vi "click_sp_coord.vi"(8 "error in (no error)":errorcluster, 10 "Panel":refnum<vi>, 11 "SubPanel in":refnum<vi>) -> (0 "error out":errorcluster, 2 "Vertical":dbl, 3 "Horizontal":dbl)   [LabVIEW 2020, in "ui-testing.lvlib"]
uses:
  ui-testing.lvlib
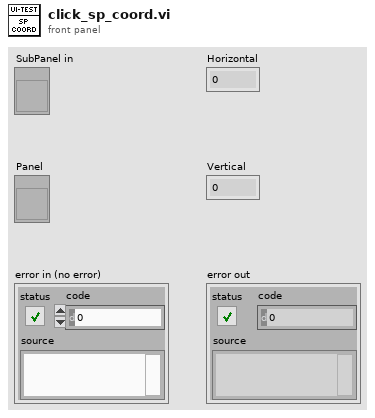
[diagram p1: front panel]
types:
  T1 = typedef "LVPositionTypeDef.ctl" = cluster{"Left":i32, "Top":i32}
  T2 = typedef "LVPointTypeDef.ctl" = cluster{"Horizontal":i16, "Vertical":i16}
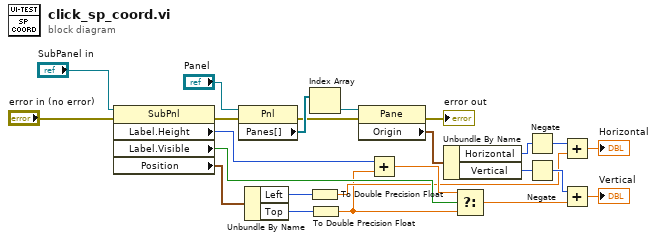
[diagram p0: block diagram]
diagram:
  n1 = property class="SubPnl"(reference="SubPanel in", error in="error in (no error)") -> (error out=w1:errorcluster, "Label.Height"=w6:u32, "Label.Visible"=w9:bool, "Position"=w11:T1)  [unwired: 1 out]
  n2 = property class="Pnl"(reference="Panel", error in=w1) -> (error out=w12:errorcluster, "Panes[]"=w13:refnum<vi>[])  [unwired: 1 out]
  n3 = Unbundle By Name(w11) -> ("Left"=w10:i32, "Top"=w8:i32)
  n4 = Index Array(array=w13) -> (element=w14:refnum<vi>)  [unwired: 1 in]
  n5 = To Double Precision Float(number=w10) -> (double precision float=w4:dbl)
  n6 = To Double Precision Float(number=w8) -> (double precision float=w3:dbl)
  n7 = property class="Pane"(reference=w14, error in=w12) -> (error out=→"error out":errorcluster, "Origin"=w15:T2)  [unwired: 1 out]
  n8 = Add(x=w6, y=w3) -> (x+y=w7:dbl)
  n9 = Unbundle By Name(w15) -> ("Horizontal"=w16:i16, "Vertical"=w19:i16)
  n10 = Select(t=w7, s=w9, f=w3) -> (s? t:f=w5:dbl)
  n11 = Negate(x=w16) -> (-x=w18:i16)
  n12 = Negate(x=w19) -> (-x=w20:i16)
  n13 = Add(x=w18, y=w4) -> (x+y=→"Horizontal":dbl)
  n14 = Add(x=w20, y=w5) -> (x+y=→"Vertical":dbl)
